vi "Serial Read Status.vi"(8 "error in (no error)":errorcluster, 11 "FW Arduino Control in":refnum<class "FW Arduino Control.lvclass">) -> (0 "error out":errorcluster, 3 "FW Arduino Control out":refnum<class "FW Arduino Control.lvclass">)   [LabVIEW 2021, in "FW Arduino Control.lvclass"]
uses:
  FW Arduino Control.lvclass
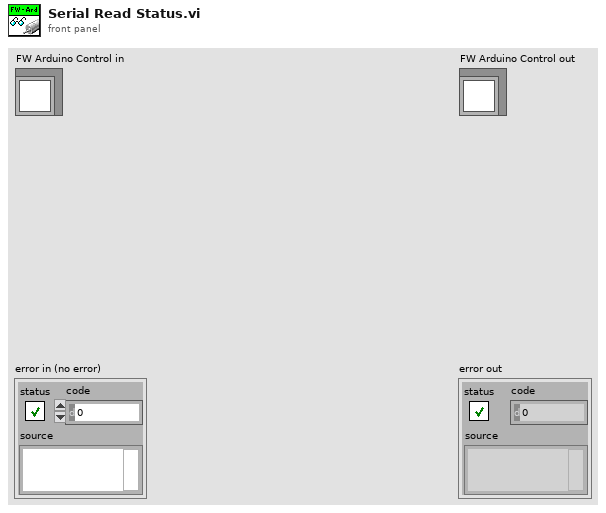
[diagram p1: front panel]
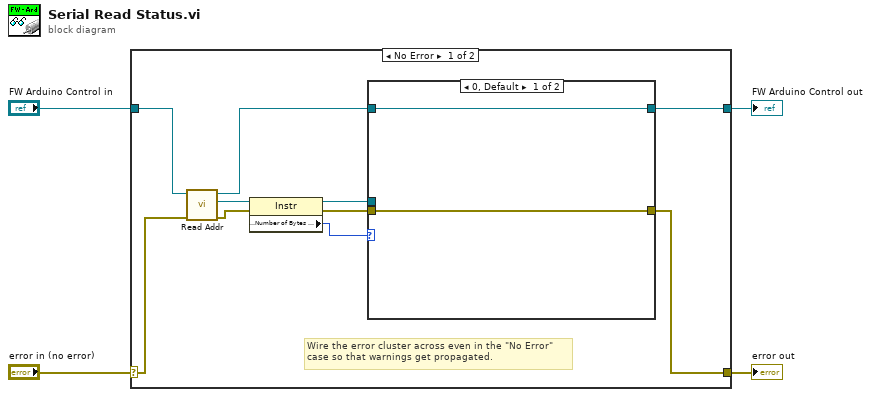
[diagram p0: block diagram]
diagram:
  n1 = case shown="No Error" "error in (no error)" {
    selector: "error in (no error)" -> [w8 w20]
    tunnel: [w5 w20] -> w3
    tunnel: [w10 w19] -> w1
    tunnel: "FW Arduino Control in" -> [w14 w19]
    frame No Error {
      # "Wire the error cluster across even in the \"No Error\"\ncase so that warnings get propagated."
      n2 = call-dynamic "Read Addr.vi"("error in (no error)"=w8, "Filter Wheel in"=w14) -> ("error out"=w7:errorcluster, "Addr"=w13:refnum<visa-resource-name>, "Filter Wheel out"=w11:refnum<class "FW Arduino Control.lvclass">)  [unwired: 7 in]
      n3 = property class="Instr"(reference=w13, error in=w7) -> (reference out=w9:refnum<visa-resource-name>, error out=w6:errorcluster, "Serial Settings:Number of Bytes at Serial Port"=w12:u32)
      n4 = case shown="0, Default" w12 {
        tunnel: w11 -> [w15 w18]
        tunnel: [w15 w18] -> w10
        tunnel: w9 -> [_ _]
        tunnel: w6 -> [w16 w17]
        tunnel: [w16 w17] -> w5
        frame 0, Default {
        }
        frame 1.. {
          # "If any bytes at port, wait for complete message."
        }
      }
    }
    frame Error {
    }
  }
  "error out" <- w3
  "FW Arduino Control out" <- w1
